vi "From JSON.vi"(7 "LVClass Serializer":refnum<class "JSONtext LVClass Serializer.lvclass">, 8 "error in (no error)":errorcluster, 10 "<JSON>":string, 11 "JSON Serializable in":refnum<class "JSON Serializable.lvclass">) -> (0 "error out":errorcluster, 3 "JSON Serializable out":refnum<class "JSON Serializable.lvclass">)   [LabVIEW 2017, in "JSON Serializable.lvclass"]
doc: "Reads data from a JSON string."
uses:
  JSON Serializable.lvclass
  <vilib>/JDP Science/JSONtext/LVClass Serializer/JSONtext LVClass Serializer.lvclass
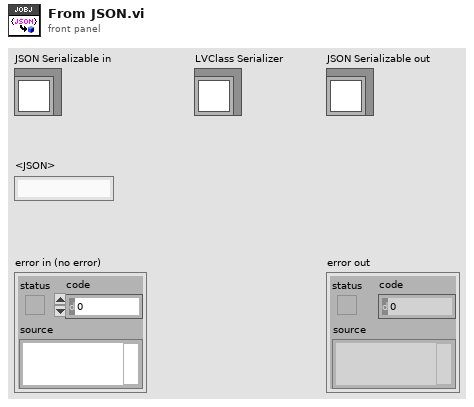
[diagram p1: front panel]
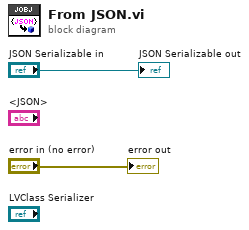
[diagram p0: block diagram]
diagram:
  "error out" <- "error in (no error)"
  "JSON Serializable out" <- "JSON Serializable in"
